vi "Linux.vi"(8 "error in (no error)":errorcluster, 10 "Font in":string, 11 "Font":refnum<vi>) -> (0 "error out":errorcluster, 2 "Font out":string)   [LabVIEW 2025]
uses:
  <vilib>/LabVIEW Icon API/lv_icon/lv_icon.lvlib
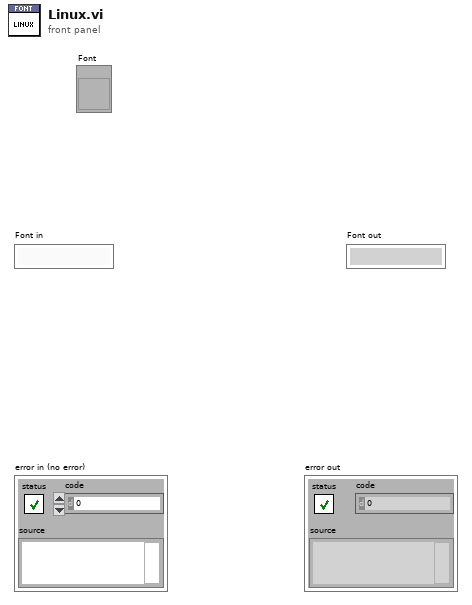
[diagram p1: front panel]
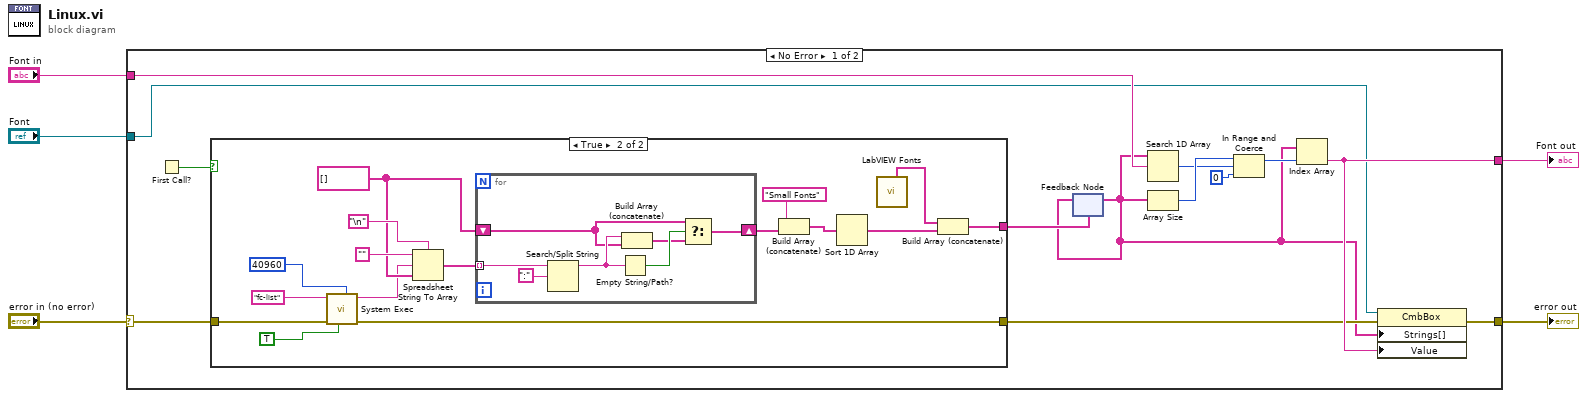
[diagram p0: block diagram]
diagram:
  n1 = case shown="No Error" "error in (no error)" {
    selector: "error in (no error)" -> [w18 w44]
    tunnel: [w17 w44] -> w4
    tunnel: "Font in" -> [w12 w43]
    tunnel: [w11 w43] -> w2
    tunnel: "Font" -> [w10 _]
    frame No Error {
      n2 = First Call?() -> (First Call?: T/F=w6:bool)
      n3 = case shown="True" w6 {
        tunnel: w18 -> [w19 w27]
        tunnel: [w19 w23] -> w9
        tunnel: [_ w22] -> w8
        frame False {
        }
        frame True {
          w29 = string[] []
          n4 = call <vilib>:"System Exec.vi"("expected output size  (4096)"=u32 40960, "run minimized? (F)"=TRUE, "error in (no error)"=w27, "command line"="fc-list") -> ("error out"=w23:errorcluster, "standard output"=w26:string)  [unwired: 3 in, 3 out]
          n5 = Spreadsheet String To Array(delimiter (Tab)="\n", format string="", spreadsheet string=w26, array type (2D Dbl)=w29) -> (array=w30:string[])
          n6 = for {
            tunnel: w30 -> [w42] mode=indexing
            shift-right: [w36] -> w28
            shift-left: w29 -> [w38]
            n7 = Search/Split String(string=w42, search string/char (-)=":") -> (substring before match=w39:string)  [unwired: 3 out]
            n8 = Empty String/Path?(string/path=w39) -> (empty?=w40:bool)
            n9 = Build Array (concatenate)(w39, w38) -> (w37:string[])
            n10 = Select(t=w38, s=w40, f=w37) -> (s? t:f=w36:string[])
          }
          n11 = Build Array (concatenate)("Small Fonts", w28) -> (w21:string[])
          n12 = Sort 1D Array(array=w21) -> (sorted array=w25:string[])
          n13 = call <vilib>:"LabVIEW Fonts.vi"() -> ("Additional Fonts"=w24:string[])  [unwired: 1 in, 10 out]
          n14 = Build Array (concatenate)(w24, w25) -> (w22:string[])
        }
      }
      n15 = feedback #1(w8) -> (w7:string[])
      n16 = feedback-in #1(w7) -> ()
      n17 = Search 1D Array(1D array=w7, element=w12) -> (index of element=w13:i32)  [unwired: 1 out]
      n18 = Array Size(array=w7) -> (size(s)=w16:i32)
      n19 = In Range and Coerce(upper limit=w16, x=w13, lower limit=0 ("x")) -> (coerced(x)=w15:i32)  [unwired: 1 out]
      n20 = Index Array(array=w7, index=w15) -> (element=w11:string)
      n21 = property class="CmbBox"(reference=w10, error in=w9, "Strings[]"=w7, "Value"=w11) -> (error out=w17:errorcluster)  [unwired: 1 out]
    }
    frame Error {
    }
  }
  "error out" <- w4
  "Font out" <- w2
